vi "Programming Assigment.vi"() -> ()   [LabVIEW 2020]
uses:
  state control.ctl
panel:
  out "Output":string
  out "Delievered":bool
  out "Credit":dbl
  out "Changes":dbl
  in  "Return Change":bool
  in  "Cluster":T1
  in  "Cancel Button":bool
  in  "10 Cents":bool
  in  "25 Cents":bool
  in  "5 Cents":bool
  # "Vending Machine"
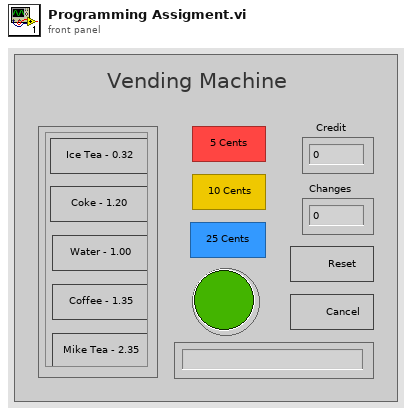
[diagram p1: front panel]
types:
  T1 = cluster{"Ice Tea":bool, "Coke":bool, "Water":bool, "Coffee":bool, "Mike Tea":bool}
  T2 = typedef "state control.ctl" = enum16{"Choose Item", "Add Money", "5 Cent", "10 Cent", "25 Cent", "Check", "Calculate"}
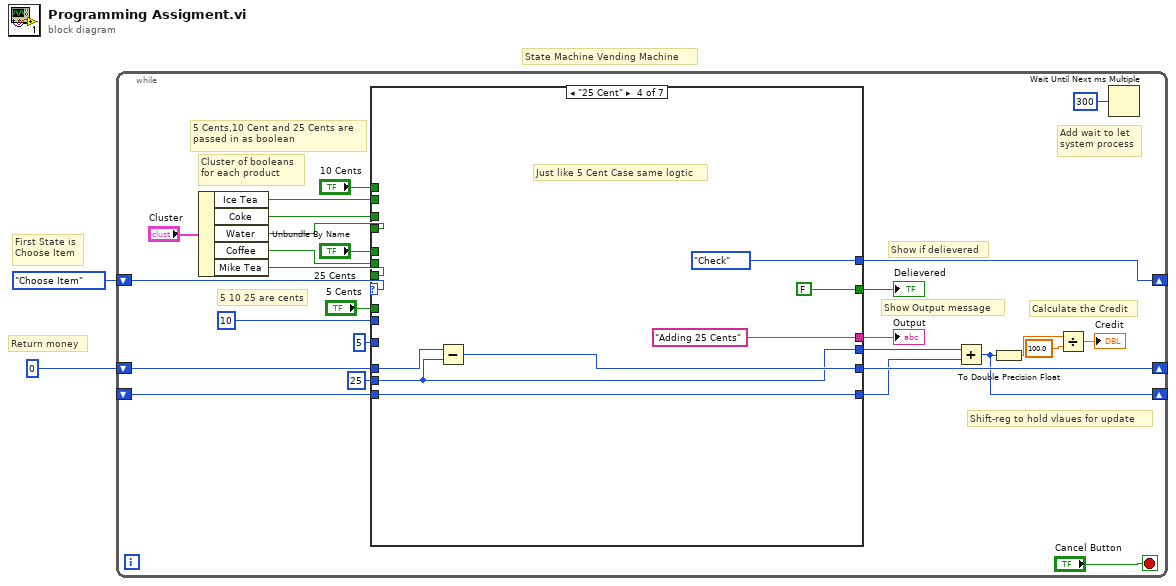
[diagram p0: block diagram]
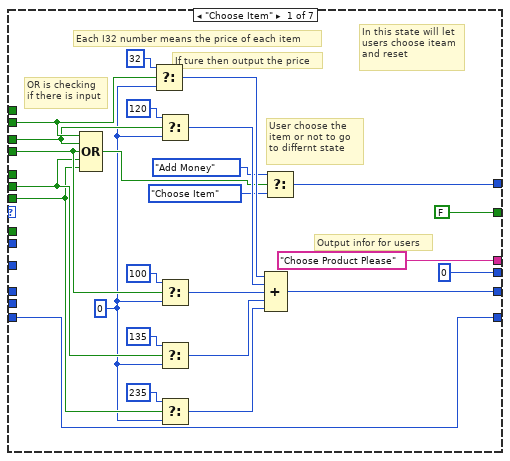
[diagram p2: hidden frame]
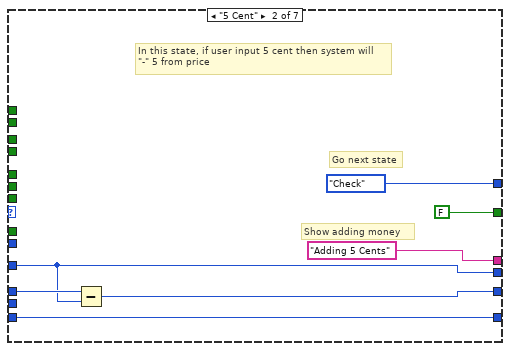
[diagram p3: hidden frame]
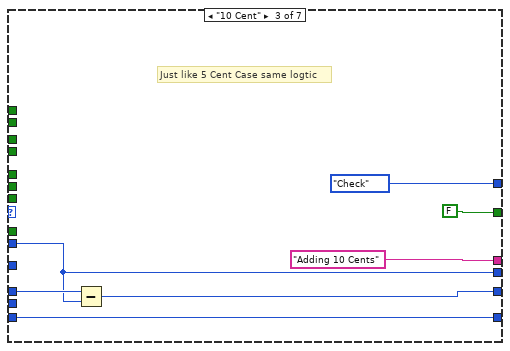
[diagram p4: hidden frame]
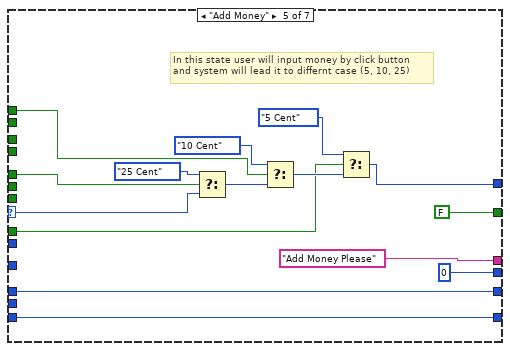
[diagram p5: hidden frame]
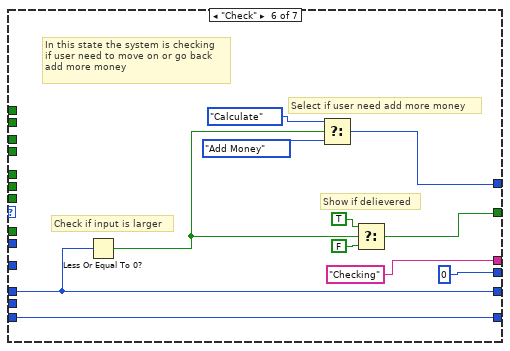
[diagram p6: hidden frame]
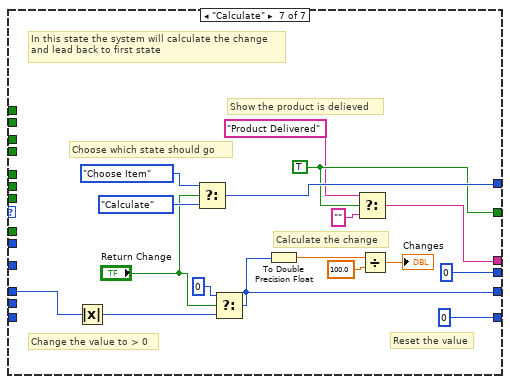
[diagram p7: hidden frame]
diagram:
  # "Return money"
  # "State Machine Vending Machine"
  # "First State is \nChoose Item"
  n1 = while {
    shift-right: [w23] -> _
    shift-left: state_control."Choose Item" -> [w24]
    shift-right: [w22] -> _
    shift-left: 0 -> [w21]
    shift-right: [w6] -> _
    shift-left: _ -> [w10]
    stop <- "Cancel Button" stop-if-true
    # "Add wait to let \nsystem process"
    # "Calculate the Credit"
    # "Show Output message"
    # "Show if delievered"
    # "Shift-reg to hold vlaues for update"
    # "5 10 25 are cents"
    # "5 Cents,10 Cent and 25 Cents are\npassed in as boolean"
    # "Cluster of booleans\nfor each product"
    n2 = Unbundle By Name("Cluster") -> ("Ice Tea"=w19:bool, "Coke"=w18:bool, "Water"=w17:bool, "Coffee"=w16:bool, "Mike Tea"=w15:bool)
    n3 = case shown="\"25 Cent\"" w24 {
      selector: w24 -> [_ _ _ _ w85 _ _]
      tunnel: [w44 w61 w68 w75 w83 w98 w103] -> w22
      tunnel: "5 Cents" -> [_ _ _ _ w80 _ _]
      tunnel: "10 Cents" -> [_ _ _ _ w82 _ _]
      tunnel: "25 Cents" -> [_ _ _ _ w81 _ _]
      tunnel: [w41 state_control."Check" state_control."Check" state_control."Check" w84 w100 w116] -> w23
      tunnel: w21 -> [_ w59 w66 w73 w83 w98 w115]
      tunnel: w19 -> [w39 _ _ _ _ _ _]
      tunnel: w18 -> [w38 _ _ _ _ _ _]
      tunnel: w17 -> [w37 _ _ _ _ _ _]
      tunnel: w16 -> [w36 _ _ _ _ _ _]
      tunnel: w15 -> [w35 _ _ _ _ _ _]
      tunnel: 5 ("y") -> [_ w56 _ _ _ _ _]
      tunnel: 10 ("y") -> [_ _ w63 _ _ _ _]
      tunnel: 25 -> [_ _ _ w71 _ _ _]
      tunnel: [FALSE FALSE FALSE FALSE FALSE w94 w111] -> w11
      tunnel: w10 -> [w33 w57 w64 w70 w78 w93 _]
      tunnel: [w33 w57 w64 w70 w78 w93 0] -> w8
      tunnel: [0 ("y") w56 w63 w71 0 ("y") 0 ("y") 0 ("y")] -> w9
      tunnel: ["Choose Product Please" "Adding 5 Cents" "Adding 10 Cents" "Adding 25 Cents" "Add Money Please" "Checking" w107] -> w7
      frame "Choose Item" {
        w30 = 0 ("f")
        # "In this state will let \nusers choose iteam\nand reset"
        # "User choose the \nitem or not to go \nto differnt state"
        # "If ture then output the price"
        # "Each I32 number means the price of each item"
        # "OR is checking\nif there is input"
        # "Output infor for users"
        n4 = Compound Arithmetic op=OR(w39, w38, w37, w36, w35) -> (w43:bool)
        n5 = Select(t=32, s=w39, f=w30) -> (s? t:f=w49:i32)
        n6 = Select(t=120, s=w38, f=w30) -> (s? t:f=w48:i32)
        n7 = Select(t=100, s=w37, f=w30) -> (s? t:f=w47:i32)
        n8 = Select(t=135, s=w36, f=w30) -> (s? t:f=w46:i32)
        n9 = Select(t=235, s=w35, f=w30) -> (s? t:f=w45:i32)
        n10 = Select(t=state_control."Add Money", s=w43, f=state_control."Choose Item") -> (s? t:f=w41:T2)
        n11 = Compound Arithmetic op=ADD(w49, w48, w47, w46, w45) -> (w44:i32)
      }
      frame "5 Cent" {
        # "Show adding money"
        # "In this state, if user input 5 cent then system will\n\"-\" 5 from price"
        # "Go next state"
        n12 = Subtract(x=w59, y=w56) -> (x-y=w61:i32)
      }
      frame "10 Cent" {
        # "Just like 5 Cent Case same logtic"
        n13 = Subtract(x=w66, y=w63) -> (x-y=w68:i32)
      }
      frame "25 Cent" {
        # "Just like 5 Cent Case same logtic"
        n14 = Subtract(x=w73, y=w71) -> (x-y=w75:i32)
      }
      frame "Add Money" {
        # "In this state user will input money by click button\nand system will lead it to differnt case (5, 10, 25)"
        n15 = Select(t=state_control."25 Cent", s=w81, f=w85) -> (s? t:f=w88:T2)
        n16 = Select(t=state_control."10 Cent", s=w82, f=w88) -> (s? t:f=w89:T2)
        n17 = Select(t=state_control."5 Cent", s=w80, f=w89) -> (s? t:f=w84:T2)
      }
      frame "Check" {
        # "In this state the system is checking\nif user need to move on or go back\nadd more money"
        # "Show if delievered"
        # "Select if user need add more money"
        # "Check if input is larger"
        n18 = Less Or Equal To 0?(x=w98) -> (x <= 0?=w97:bool)
        n19 = Select(t=state_control."Calculate", s=w97, f=state_control."Add Money") -> (s? t:f=w100:T2)
        n20 = Select(t=TRUE, s=w97, f=FALSE) -> (s? t:f=w94:bool)
      }
      frame "Calculate" {
        w111 = TRUE
        # "Change the value to > 0"
        # "Reset the value"
        # "Calculate the change"
        # "Choose which state should go"
        # "Show the product is delieved"
        # "In this state the system will calculate the change\nand lead back to first state"
        n21 = Absolute Value(x=w115) -> (abs(x)=w113:i32)
        n22 = Select(t=state_control."Choose Item", s="Return Change", f=state_control."Calculate") -> (s? t:f=w116:T2)
        n23 = Select(t=0, s="Return Change", f=w113) -> (s? t:f=w103:i32)
        n24 = To Double Precision Float(number=w103) -> (double precision float=w105:dbl)
        n25 = Select(t="Product Delivered", s=w111, f="") -> (s? t:f=w107:string)
        n26 = Divide(x=w105, y=100.0) -> (x/y=→"Changes":dbl)
      }
    }
    "Delievered" <- w11
    "Output" <- w7
    n27 = Add(x=w9, y=w8) -> (x+y=w6:i32)
    n28 = To Double Precision Float(number=w6) -> (double precision float=w5:dbl)
    n29 = Divide(x=w5, y=100.0) -> (x/y=→"Credit":dbl)
    n30 = Wait Until Next ms Multiple(millisecond multiple=u32 300 ("milliseconds to wait")) -> ()  [unwired: 1 out]
  }
